vi "Check bytes at port.vi"(8 "error in (no error)":errorcluster, 11 "ArduinoAIReal in":refnum<class "Arduino.lvclass">) -> (0 "error out":errorcluster, 1 "Bytes available":bool, 2 "Number of Bytes at Serial Port":u32, 3 "ArduinoAIReal out":refnum<class "Arduino.lvclass">)   [LabVIEW 2020, in "Arduino.lvlib" / "Arduino.lvclass"]
uses:
  Arduino.lvclass
  Arduino.lvclass/Arduino.ctl
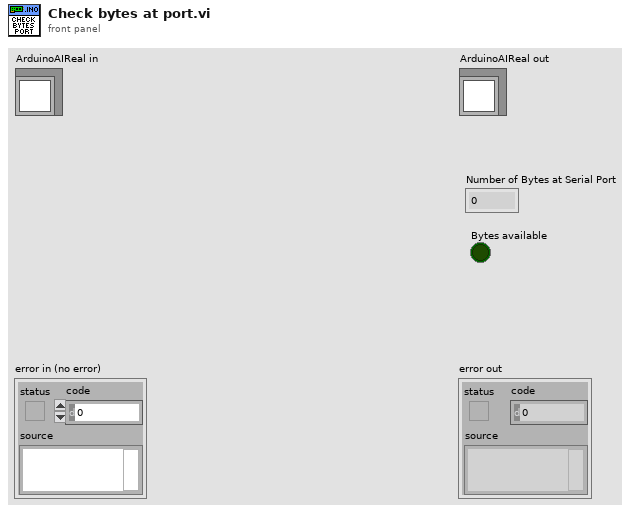
[diagram p1: front panel]
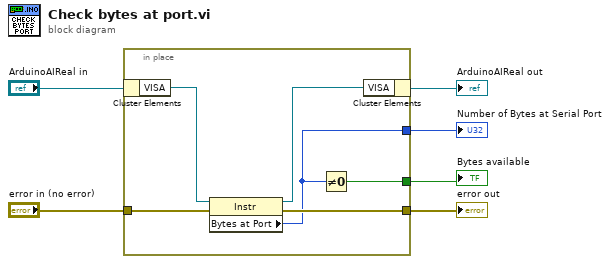
[diagram p0: block diagram]
diagram:
  n1 = in-place {
    in-place-border: "error in (no error)" -> [w12]
    in-place-border: [w11] -> w5
    in-place-border: [w10] -> w4
    in-place-border: [w9] -> w3
    n2 = in-place-cluster #1("ArduinoAIReal in") -> ("VISA"=w8:refnum<visa-resource-name>)
    n3 = property class="Instr"(reference=w8, error in=w12) -> (reference out=w7:refnum<visa-resource-name>, error out=w11:errorcluster, "Bytes at Port"=w10:u32)
    n4 = Not Equal To 0?(x=w10) -> (x != 0?=w9:bool)
    n5 = in-place-cluster #1("VISA"=w7) -> (→"ArduinoAIReal out":refnum<class "Arduino.lvclass">)
  }
  "error out" <- w5
  "Number of Bytes at Serial Port" <- w4
  "Bytes available" <- w3
